vi "call handlers.vi"(7 "Handlers":string[](array[string])=["Calibration", "Measurement", "Home", "Laser", "Motor", "File", "Template"], 8 "error in (no error)":errorcluster, 10 "Server Variables":T1 {"Energy Levels"."E1" format="%_6g"; "Phases"."ExtTriggerDelay" format="%.3g"}, 11 "HTTP Request in":T7) -> (0 "error out":errorcluster, 2 "Server Variables":T1 {"Energy Levels"."E1" format="%_6g"; "Phases"."ExtTriggerDelay" format="%.3g"}, 3 "HTTP Request out":T7)   [LabVIEW 2011]
uses:
  http_request_response.ctl
  http_request.ctl
  http_field.ctl
  http_response.ctl
  template_field.ctl
  template_field_type.ctl
  Server Variables.ctl
  Phase Parameters.ctl
  Phase Mode.ctl
  Energy Level_.ctl
  Measurement Parameters.ctl
  Results.ctl
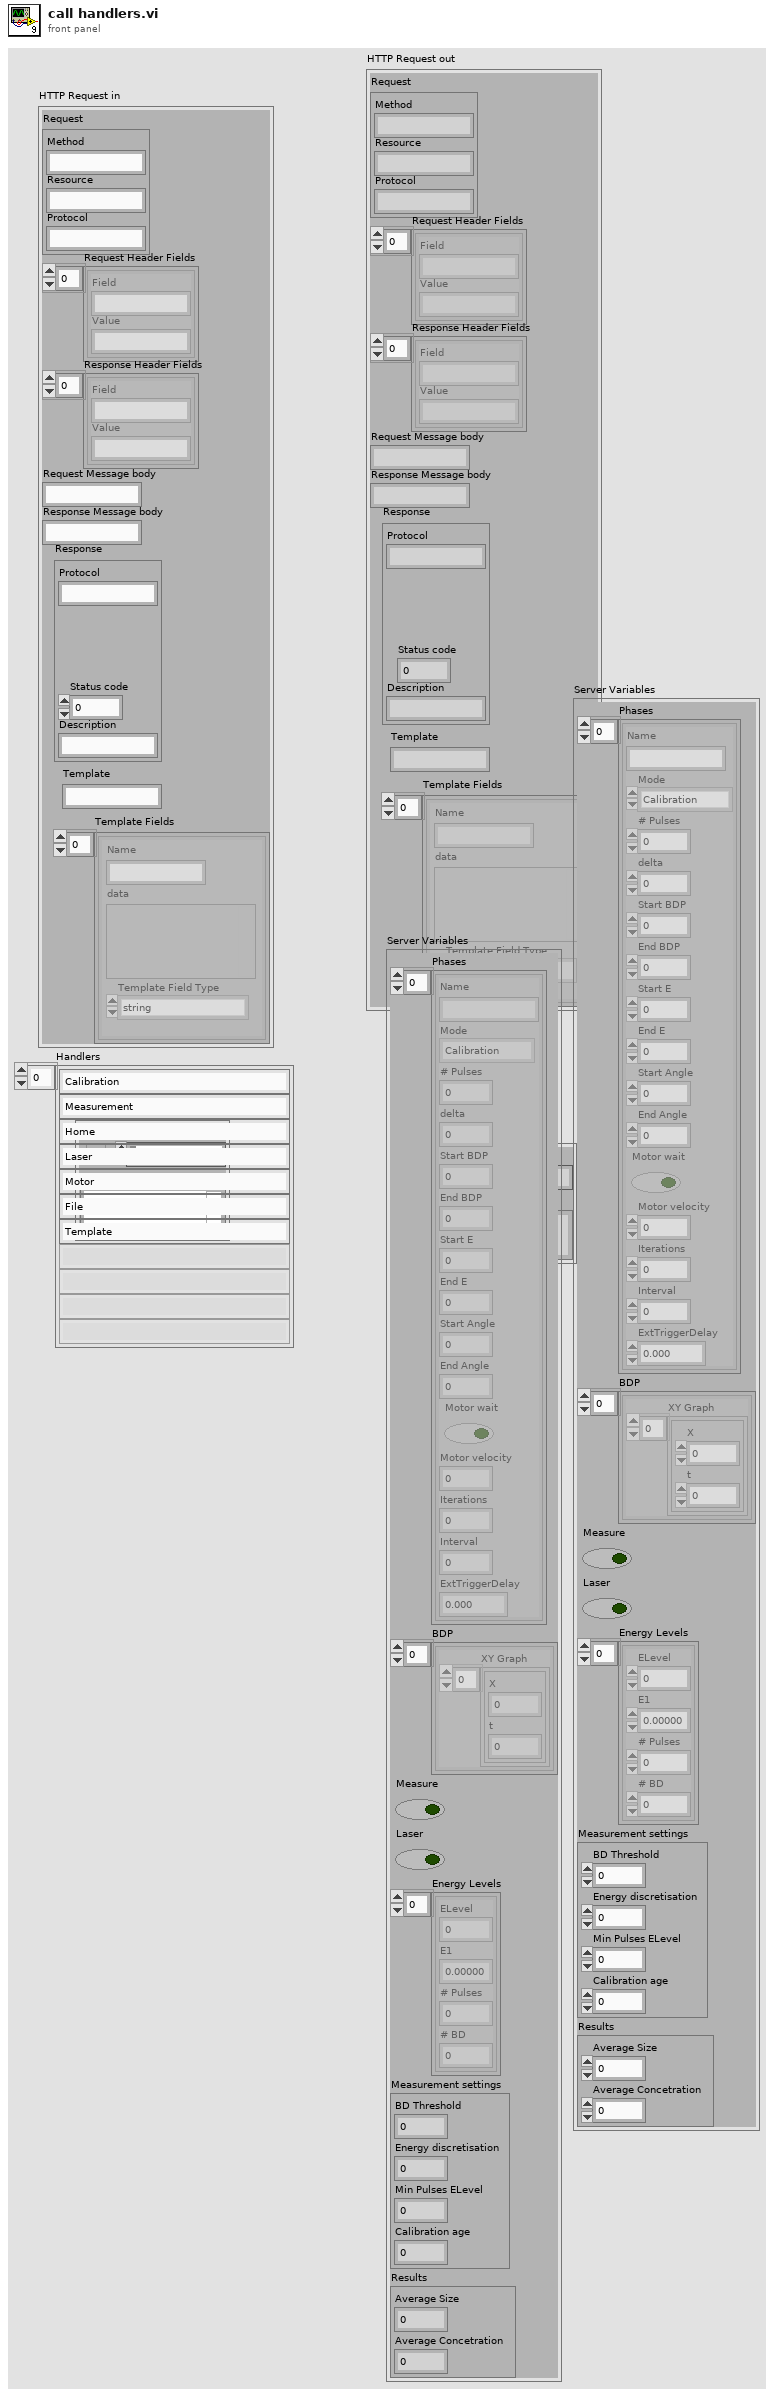
[diagram p1: front panel]
types:
  T1 = typedef "Server Variables.ctl" = cluster{"Phases":T2[], "BDP":cluster{"XY Graph":cluster{"X":dbl, "t":dbl}[]}[], "Measure":bool, "Laser":bool, "Energy Levels":T4[], "Measurement settings":T5, "Results":T6}
  T2 = typedef "Phase Parameters.ctl" = cluster{"Name":string, "Mode":T3, "# Pulses":u32, "delta":dbl, "Start BDP":dbl, "End BDP":dbl, "Start E":dbl, "End E":dbl, "Start Angle":dbl, "End Angle":dbl, "Motor wait":bool, "Motor velocity":dbl, "Iterations":dbl, "Interval":dbl, "ExtTriggerDelay":dbl}
  T3 = typedef "Phase Mode.ctl" = enum16{"Calibration", "Linear", "BDP-Fit", "Raw"}
  T4 = typedef "Energy Level_.ctl" = cluster{"ELevel":dbl, "E1":dbl, "# Pulses":i32, "# BD":i32}
  T5 = typedef "Measurement Parameters.ctl" = cluster{"BD Threshold":dbl, "Energy discretisation":i32, "Min Pulses ELevel":i32, "Calibration age":i32}
  T6 = typedef "Results.ctl" = cluster{"Average Size":dbl, "Average Concetration":dbl}
  T7 = typedef "http_request_response.ctl" = cluster{"Request":T8, "Request Header Fields":T9[], "Response Header Fields":T9[], "Request Message body":string, "Response Message body":string, "Response":T10, "Template":string, "Template Fields":T11[]}
  T8 = typedef "http_request.ctl" = cluster{"Method":string, "Resource":string, "Protocol":string}
  T9 = typedef "http_field.ctl" = cluster{"Field":string, "Value":string}
  T10 = typedef "http_response.ctl" = cluster{"Protocol":string, "Status code":dbl, "Description":string}
  T11 = typedef "template_field.ctl" = cluster{"Name":string, "Template Field Type":T12, "data":variant}
  T12 = typedef "template_field_type.ctl" = enum16{"string", "string array", "number", "number array", "cluster", "cluster array"}
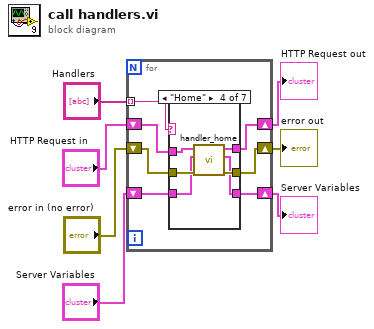
[diagram p0: block diagram]
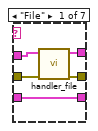
[diagram p2: hidden frame]
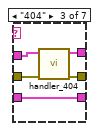
[diagram p4: hidden frame]
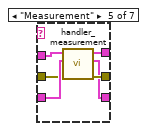
[diagram p5: hidden frame]
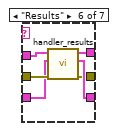
[diagram p6: hidden frame]
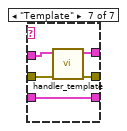
[diagram p7: hidden frame]
diagram:
  n1 = for {
    shift-right: [w8] -> w7
    shift-left: "HTTP Request in" -> [w11]
    shift-right: [w13] -> w6
    shift-left: "error in (no error)" -> [w12]
    tunnel: "Handlers" -> [w14] mode=indexing
    shift-right: [w9] -> w1
    shift-left: "Server Variables" -> [w10]
    n2 = case shown="\"Home\"" w14 {
      tunnel: [w16 w22 w25 w32 w34 w45 w47] -> w8
      tunnel: w11 -> [w19 w22 w27 w33 w39 w41 w50]
      tunnel: [w17 w21 w24 w31 w36 w43 w48] -> w13
      tunnel: w12 -> [w18 w21 w26 w30 w37 w42 w49]
      tunnel: w10 -> [w15 w20 w23 w29 w38 w40 w46]
      tunnel: [w15 w20 w23 w28 w35 w44 w46] -> w9
      frame "File" {
        n3 = call "handler_file.vi"("error in (no error)"=w18, "HTTP Request"=w19) -> ("error out"=w17:errorcluster, "HTTP Request out"=w16:T7)  [unwired: 7 in, 1 out]
      }
      frame Default {
      }
      frame "404" {
        n4 = call "handler_404.vi"("error in (no error)"=w26, "HTTP Request in"=w27) -> ("error out"=w24:errorcluster, "HTTP Request out"=w25:T7)  [unwired: 8 in]
      }
      frame "Home" {
        n5 = call "handler_home.vi"("error in (no error)"=w30, "Server Variables"=w29, "HTTP Request in"=w33) -> ("error out"=w31:errorcluster, "Server Variables"=w28:T1, "HTTP Request out"=w32:T7)  [unwired: 6 in]
      }
      frame "Measurement" {
        n6 = call "handler_measurement.vi"("error in (no error)"=w37, "Server Variables"=w38, "HTTP Request in"=w39) -> ("error out"=w36:errorcluster, "Server Variables"=w35:T1, "HTTP Request out"=w34:T7)  [unwired: 6 in]
      }
      frame "Results" {
        n7 = call "handler_results.vi"("error in (no error)"=w42, "Server Variables"=w40, "HTTP Request in"=w41) -> ("error out"=w43:errorcluster, "Server Variables"=w44:T1, "HTTP Request out"=w45:T7)  [unwired: 6 in]
      }
      frame "Template" {
        n8 = call "handler_template.vi"("error in (no error)"=w49, "HTTP Request in"=w50) -> ("error out"=w48:errorcluster, "HTTP Request out"=w47:T7)  [unwired: 7 in, 1 out]
      }
    }
  }
  "HTTP Request out" <- w7
  "error out" <- w6
  "Server Variables" <- w1
